vi "Initialize.vi"(4 "error in (no error)":errorcluster, 5 "Default setup (True)":bool=TRUE, 6 "ID Query (True)":bool=TRUE, 7 "VISA resource name":refnum<visa-resource-name>) -> (0 "error out":errorcluster, 1 "VISA resource name out":refnum<visa-resource-name>)   [LabVIEW 2014, in "GP22_TDC_Arduinoed.lvlib"]
doc: "Establishes communication with the instrument and optionally performs an instrument identification query and/or an instrument reset. It also places the instrument in a default state needed for other instrument driver operations. Therefore, call this VI before calling other instrument driver VIs for this instrument. Generally, you need to call the <b>Initialize</b> VI only once at the beginning of an application."
uses:
  GP22_TDC_Arduinoed.lvlib
panel:
  in  "Expected ID":string="GP22_DRIVER - 0.6"
  # "(c) 2014 <Enter Company Name Here>.  ALL RIGHTS RESERVED."
  # "EDIT: Change control description to remove example text for buses not supported."
  # "EDIT: Serial settings must match those on the physical instrument.  Review user's manual to determine the correct Flow Control protocol for the instrument.  \"None\" is the least robust option for this setting, and could lead to unreliable data transmission."
  # "EDIT: If your instrument does not support ID query or Reset, remove the ID Query or Reset control from the front panel and delete the case structure with the ID Query or Reset code from the block diagram."
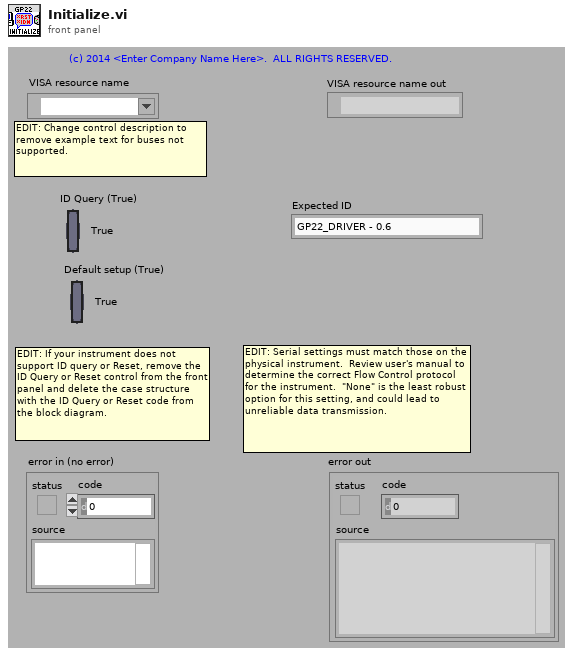
[diagram p1: front panel]
types:
  T1 = cluster{"Baud Rate":u32, "Parity":u16, "Data Bits":u16, "Stop Bits":u16, "Flow Control":u16}
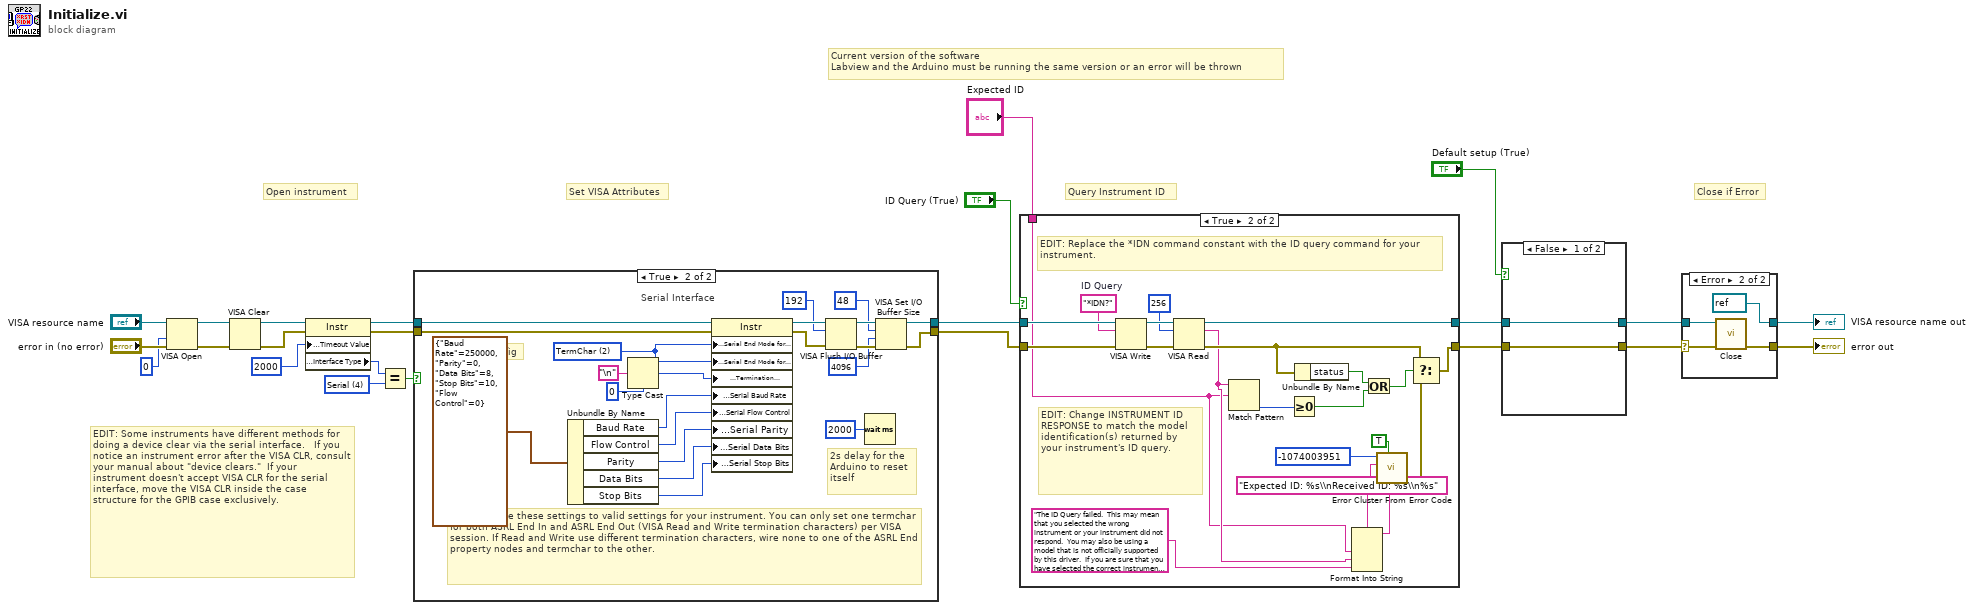
[diagram p0: block diagram]
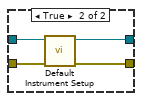
[diagram p2: hidden frame]
diagram:
  w12 = u16 4 items=["GPIB"=1, "VXI"=2, "GPIB-VXI"=3, "Serial"=4, "PXI"=5, "TCPIP"=6, "USB"=7] ("Interface Information:Interface Type")
  # "Current version of the software\nLabview and the Arduino must be running the same version or an error will be thrown"
  # "EDIT: Some instruments have different methods for doing a device clear via the serial interface.   If you notice an instrument error after the VISA CLR, consult your manual about \"device clears.\"  If your instrument doesn't accept VISA CLR for the serial interface, move the VISA CLR inside the case  structure for the GPIB case exclusively."
  # "Set VISA Attributes"
  # "Close if Error"
  # "Query Instrument ID"
  # "Open instrument"
  n1 = VISA Open(access mode=u32 0, error in (no error)="error in (no error)", VISA resource name="VISA resource name") -> (VISA resource name=w10:refnum<visa-resource-name>, error out=w9:errorcluster)  [unwired: 2 in]
  n2 = VISA Clear(VISA resource name=w10, error in (no error)=w9) -> (VISA resource name out=w8:refnum<visa-resource-name>, error out=w7:errorcluster)
  n3 = property class="Instr"(reference=w8, error in=w7, "General Settings:Timeout Value"=u32 2000) -> (reference out=w15:refnum<visa-resource-name>, error out=w14:errorcluster, "Interface Information:Interface Type"=w19:u16)
  n4 = Equal?(x=w19, y=w12) -> (x = y?=w13:bool)
  n5 = case shown="True" w13 {
    tunnel: [w25 w45] -> w17
    tunnel: [w26 w42] -> w16
    tunnel: w15 -> [w25 w47]
    tunnel: w14 -> [w26 w48]
    frame False {
      # "EDIT: Remove interfaces not supported by your instrument."
      # "GPIB, TCP/IP, and USB Interface"
    }
    frame True {
      w35 = u16 2 items=["None", "LastBit", "TermChar"] ("Serial Settings:Serial End Mode for Reads")
      # "2s delay for the\nArduino to reset\nitself"
      # "Serial config"
      # "EDIT: Change these settings to valid settings for your instrument. You can only set one termchar for both ASRL End In and ASRL End Out (VISA Read and Write termination characters) per VISA session. If Read and Write use different termination characters, wire none to one of the ASRL End property nodes and termchar to the other."
      # "Serial Interface"
      n6 = Unbundle By Name(T1 {"Baud Rate"=250000, "Parity"=0, "Data Bits"=8, "Stop Bits"=10, "Flow Control"=0} ("Serial Configuration")) -> ("Baud Rate"=w33:u32, "Flow Control"=w29:u16, "Parity"=w31:u16, "Data Bits"=w32:u16, "Stop Bits"=w28:u16)
      n7 = Type Cast(type=u8 0, x="\n" ("Line Feed Constant")) -> (*(type *) &x=w34:u8)
      n8 = property class="Instr"(reference=w47, error in=w48, "Serial Settings:Serial End Mode for Reads"=w35, "Serial Settings:Serial End Mode for Writes"=w35, "Message Based Settings:Termination Character"=w34, "Serial Settings:Serial Baud Rate"=w33, "Serial Settings:Serial Flow Control"=w29, "Serial Settings:Serial Parity"=w31, "Serial Settings:Serial Data Bits"=w32, "Serial Settings:Serial Stop Bits"=w28) -> (reference out=w41:refnum<visa-resource-name>, error out=w44:errorcluster)
      n9 = VISA Flush I/O Buffer(VISA resource name=w41, mask (16)=u16 192, error in (no error)=w44) -> (VISA resource name out=w46:refnum<visa-resource-name>, error out=w43:errorcluster)
      n10 = Wait (ms)(milliseconds to wait=u32 2000) -> ()  [unwired: 1 out]
      n11 = VISA Set I/O Buffer Size(VISA resource name=w46, mask (16)=u16 48, size (4096)=u32 4096 ("size (0)"), error in (no error)=w43) -> (VISA resource name out=w45:refnum<visa-resource-name>, error out=w42:errorcluster)
    }
  }
  n12 = case shown="True" "ID Query (True)" {
    tunnel: [w49 w71] -> w23
    tunnel: [w50 w68] -> w24
    tunnel: w17 -> [w50 w69]
    tunnel: w16 -> [w49 w70]
    tunnel: "Expected ID" -> [_ w52]
    frame False {
    }
    frame True {
      w64 = "*IDN?"  # ID Query
      # "EDIT: Replace the *IDN command constant with the ID query command for your instrument."
      # "EDIT: Change INSTRUMENT ID RESPONSE to match the model identification(s) returned by your instrument's ID query."
      n13 = VISA Write(VISA resource name=w69, write buffer=w64, error in (no error)=w70) -> (VISA resource name out=w67:refnum<visa-resource-name>, error out=w66:errorcluster)  [unwired: 1 out]
      n14 = VISA Read(VISA resource name=w67, byte count=u32 256, error in (no error)=w66) -> (VISA resource name out=w68:refnum<visa-resource-name>, read buffer=w53:string, error out=w59:errorcluster)  [unwired: 1 out]
      n15 = Match Pattern(string=w53, regular expression=w52) -> (offset past match=w60:i32)  [unwired: 1 in, 3 out]
      n16 = Greater Or Equal To 0?(x=w60) -> (x >= 0?=w57:bool)
      n17 = Unbundle By Name(w59) -> ("status"=w58:bool)
      n18 = Format Into String(format string="Expected ID: %s\\nReceived ID: %s\\n%s", w52, w53, "The ID Query failed.  This may mean that you selected the wrong instrument or your instrument did not respond.  You may also be using a model that is not officially supported by this driver.  If you are sure that you have selected the correct instrument and it is responding, try disabling the ID Query." ("Source (VI Name)")) -> (resulting string=w55:string)  [unwired: 2 in, 1 out]
      n19 = Or(x=w58, y=w57) -> (x .or. y?=w56:bool)
      n20 = call <vilib>:"Error Cluster From Error Code.vi"("show call chain? (False)"=TRUE, "error message (\"\")"=w55, "error code (0)"=-1074003951 ("Code")) -> ("error out"=w63:errorcluster)  [unwired: 6 in]
      n21 = Select(t=w59, s=w56, f=w63) -> (s? t:f=w71:errorcluster)
    }
  }
  n22 = case shown="False" "Default setup (True)" {
    tunnel: w24 -> [w73 w77]
    tunnel: w23 -> [w72 w76]
    tunnel: [w73 w75] -> w4
    tunnel: [w72 w74] -> w3
    frame False {
    }
    frame True {
      n23 = call "Default Instrument Setup.vi"("error in (no error)"=w76, "VISA resource name"=w77) -> ("error out"=w74:errorcluster, "VISA resource name out"=w75:refnum<visa-resource-name>)  [unwired: 8 in]
    }
  }
  n24 = case shown="Error" w3 {
    selector: w3 -> [w78 w81]
    tunnel: w4 -> [w79 w82]
    tunnel: [w79 refnum<visa-resource-name> refnum ("VISA resource name out")] -> w6
    tunnel: [w78 w83] -> w5
    frame No Error {
    }
    frame Error {
      n25 = call "Close.vi"("error in (no error)"=w81, "VISA resource name"=w82) -> ("error out"=w83:errorcluster)  [unwired: 9 in]
    }
  }
  "VISA resource name out" <- w6
  "error out" <- w5
